vi "build refresh token URI.vi"(8 "error in (no error)":errorcluster, 11 "Oauth2.Salesforce in":refnum<class "Oauth2.Salesforce.lvclass">) -> (0 "error out":errorcluster, 2 "Refresh Token Request URI":string, 3 "Oauth2.Salesforce":refnum<class "Oauth2.Salesforce.lvclass">)   [LabVIEW 2017]
uses:
  Oauth2.Salesforce.lvclass/Oauth2.Salesforce.ctl
  Oauth2.Salesforce.lvclass
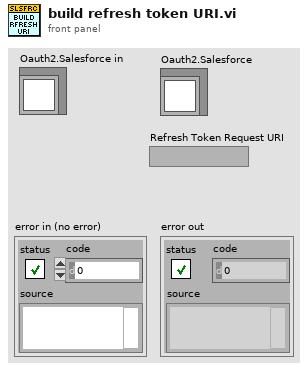
[diagram p1: front panel]
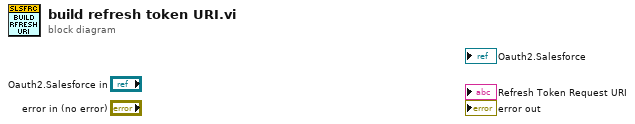
[diagram p0: block diagram]
diagram:
